vi "Evaluate Targets for Shooting.vi"(8 "Distance Method":u16(ring)=2 items=["Default", "Center Calculations", "Hybrid"], 9 "Camera Distance\nfrom Ground (in)":dbl, 10 "Maximum Shooting Distance":dbl, 11 "More Detection":T1(array[cluster])) -> (3 "Shootable":bool)   [LabVIEW 2015]
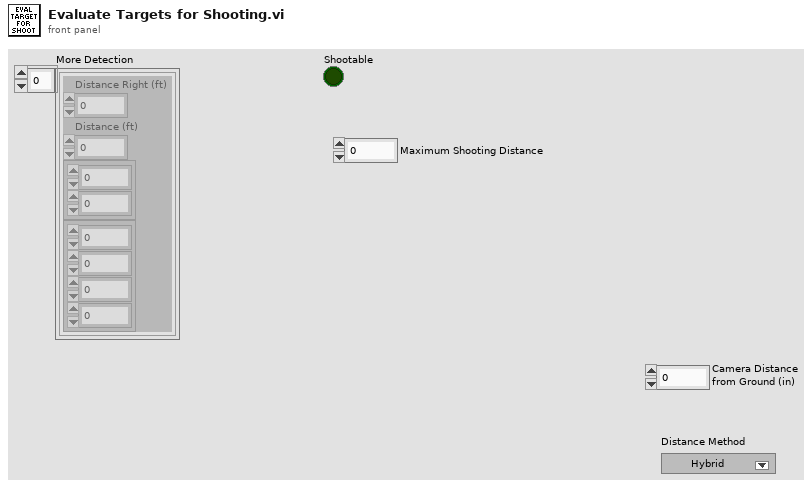
[diagram p1: front panel]
types:
  T1 = cluster{"Distance Right (ft)":dbl, "Distance (ft)":dbl, cluster{dbl, dbl}, cluster{dbl, dbl, dbl, dbl}}[]
  T2 = cluster{"Distance Right (ft)":dbl, "Distance (ft)":dbl, cluster{dbl, dbl}, cluster{dbl, dbl, dbl, dbl}}
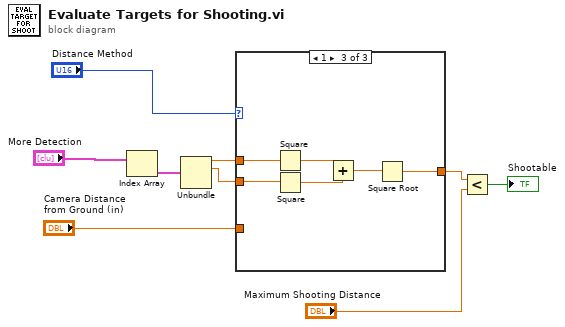
[diagram p0: block diagram]
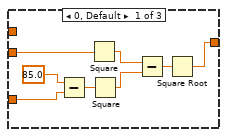
[diagram p2: hidden frame]
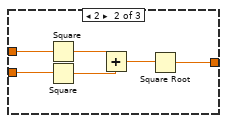
[diagram p3: hidden frame]
diagram:
  n1 = Index Array(array="More Detection") -> (element=w7:T2)  [unwired: 1 in]
  n2 = Unbundle(w7) -> ("Distance Right (ft)"=w6:dbl, "Distance (ft)"=w5:dbl)  [unwired: 2 out]
  n3 = case shown="1" "Distance Method" {
    tunnel: w6 -> [_ w20 w26]
    tunnel: w5 -> [w17 w19 w25]
    tunnel: "Camera Distance\nfrom Ground (in)" -> [w14 _ _]
    tunnel: [w10 w18 w24] -> w3
    frame 0, Default {
      n4 = Subtract(x=85.0, y=w14) -> (x-y=w13:dbl)
      n5 = Square(x=w17) -> (x^2=w16:dbl)
      n6 = Square(x=w13) -> (x^2=w12:dbl)
      n7 = Subtract(x=w16, y=w12) -> (x-y=w11:dbl)
      n8 = Square Root(x=w11) -> (sqrt(x)=w10:dbl)
    }
    frame 2 {
      n9 = Square(x=w20) -> (x^2=w23:dbl)
      n10 = Square(x=w19) -> (x^2=w22:dbl)
      n11 = Add(x=w23, y=w22) -> (x+y=w21:dbl)
      n12 = Square Root(x=w21) -> (sqrt(x)=w18:dbl)
    }
    frame 1 {
      n13 = Square(x=w26) -> (x^2=w29:dbl)
      n14 = Square(x=w25) -> (x^2=w28:dbl)
      n15 = Add(x=w29, y=w28) -> (x+y=w27:dbl)
      n16 = Square Root(x=w27) -> (sqrt(x)=w24:dbl)
    }
  }
  n17 = Less?(x=w3, y="Maximum Shooting Distance") -> (x < y?=→"Shootable":bool)
